vi "Chad Magic Voodoo.vi"() -> ()   [LabVIEW 2016]
panel:
  out "W trigger Y":dbl
  out "C trigger Y":dbl
  out "R trigger Y":dbl
  in  "Window Bead Trigger heights":dbl[](array[numeric])
  in  "Robot Bead Trigger heights":dbl[](array[numeric])
  in  "Center Bead Trigger heights":dbl[](array[numeric])
  out "Shutter Open":bool
  in  "Distance from\n Bead Height":dbl
  out "Recommended % Change\n in Wire Feed 1":dbl
  in  "base path":path=path "C:/Users/Mark/Desktop/BeadScan"
  in  "Write Code":bool
  out "Bead3 Size":i32
  out "Bead2 Size":i32
  out "Bead1 Size":i32
  in  "Tab Control":T1(tab)
  in  "Mark Target Bead Height":bool
  out "All Beads":cluster{dbl[], dbl[]}[](graph)
  out "Target Bead Height":dbl
  in  "Set Trigger Offset":dbl
  in  "Center Bead Corrections":dbl[](array[numeric])
  in  "Center Bead Trigger Positions":dbl[](array[numeric])
  out "Center Bead #1":cluster{dbl[], dbl[]}[](graph)
  out "Center Bead Trigger":dbl
  in  "Set Trigger Center":bool
  in  "Undo":bool
  out "Difference From Bead Height Setpoint C":dbl
  out "Recommended % Change\n in Wire Feed C":dbl
  out "Minus 5- Too lazy to math":dbl
  in  "Set Trigger Offset 2":dbl
  out "Robot Bead #2":cluster{dbl[], dbl[]}[](graph)
  in  "Robot Bead Trigger Positions":dbl[](array[numeric])
  in  "Robot Bead Corrections":dbl[](array[numeric])
  out "Robot Bead Trigger":dbl
  in  "Set Trigger Robot":bool
  in  "Undo":bool
  out "Difference From Bead Height Setpoint R":dbl
  out "Recommended % Change\n in Wire Feed R":dbl
  in  "Set Trigger Offset 3":dbl
  out "Window Bead #3":cluster{dbl[], dbl[]}[](graph)
  in  "Window Bead Trigger Positions":dbl[](array[numeric])
  in  "Window Bead Corrections":dbl[](array[numeric])
  out "Window Bead Trigger":dbl
  in  "Set Trigger Window":bool
  in  "Undo":bool
  out "Difference From Bead Height Setpoint W":dbl
  out "Recommended % Change\n in Wire Feed W":dbl
  in  "stop":bool
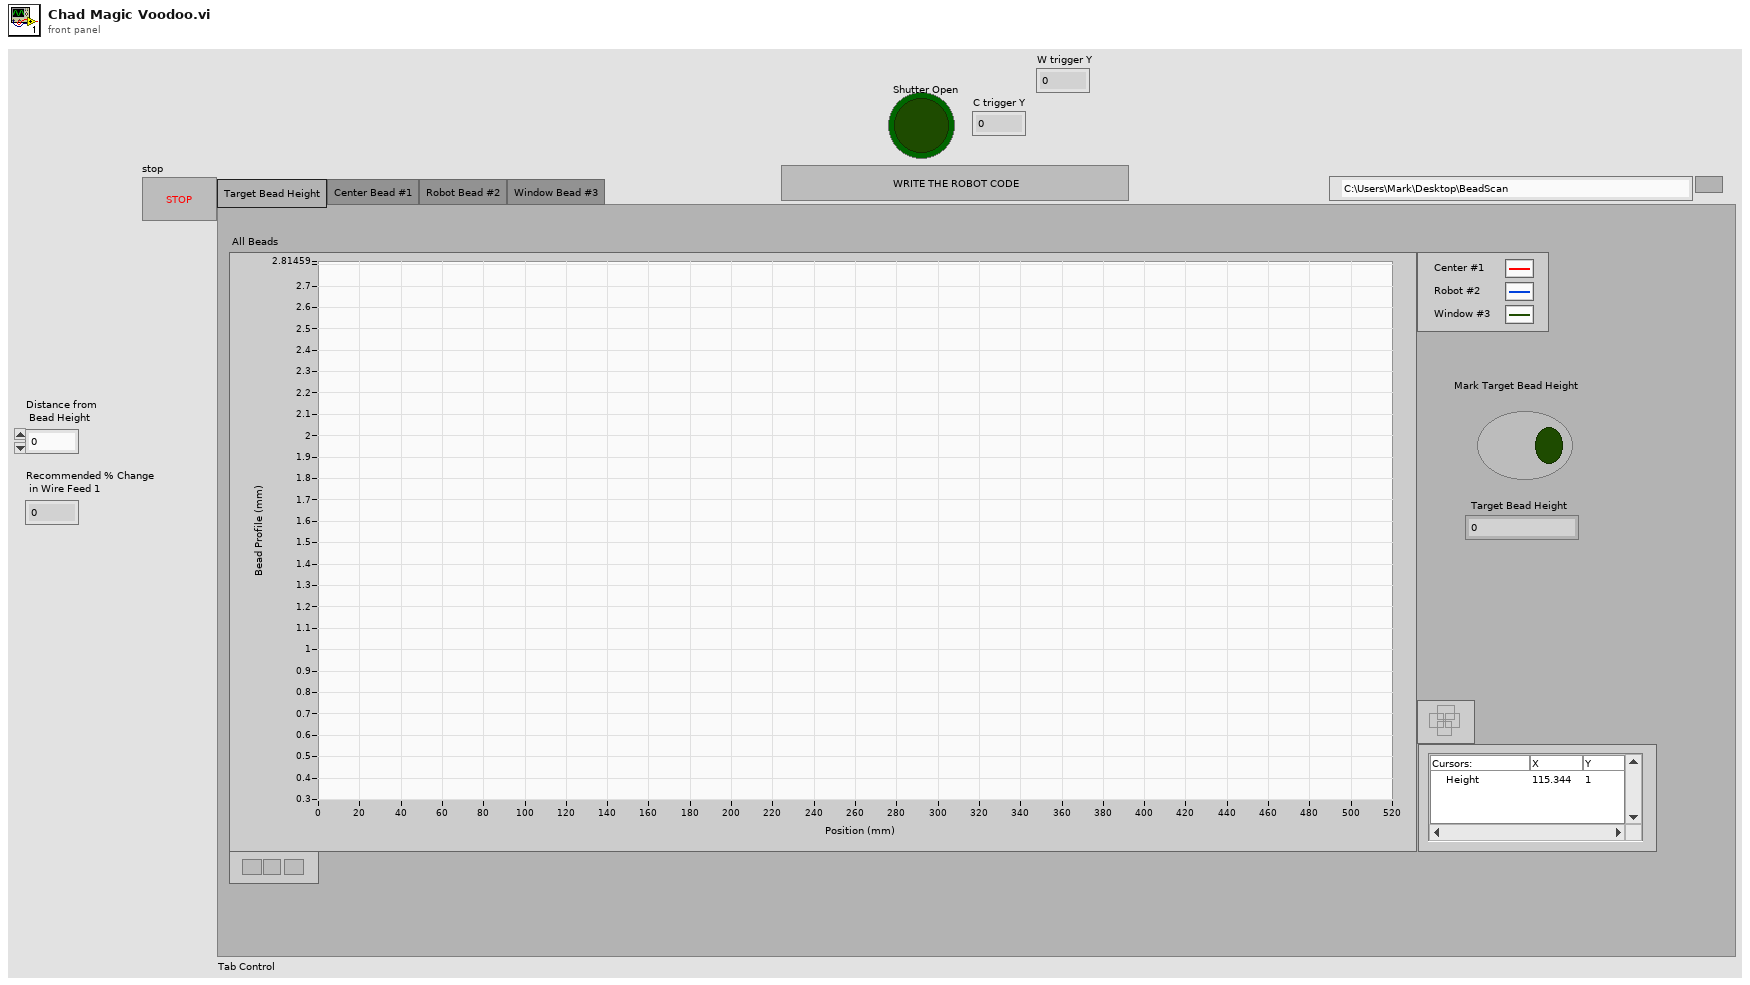
[diagram p1: front panel]
types:
  T1 = enum32{"Target Bead Height", "Center Bead #1", "Robot Bead #2", "Window Bead #3"}
  T2 = enum16{"open", "replace", "create", "open or create", "replace or create", "replace or create with confirmation"}
  T3 = cluster{"[0]":cluster{dbl[], dbl[]}, "[1]":cluster{dbl[], dbl[]}, "[2]":cluster{dbl[], dbl[]}}
  T4 = cluster{dbl[], "Center Bead Trigger heights":dbl[]}
  T5 = cluster{dbl[], "Window Bead Trigger heights":dbl[]}
  T6 = cluster{dbl[], "Robot Bead Trigger heights":dbl[]}
  T7 = cluster{dbl[], "Center Bead Trigger heights":dbl[]}[]
  T8 = cluster{dbl[], "Robot Bead Trigger heights":dbl[]}[]
  T9 = cluster{dbl[], "Window Bead Trigger heights":dbl[]}[]
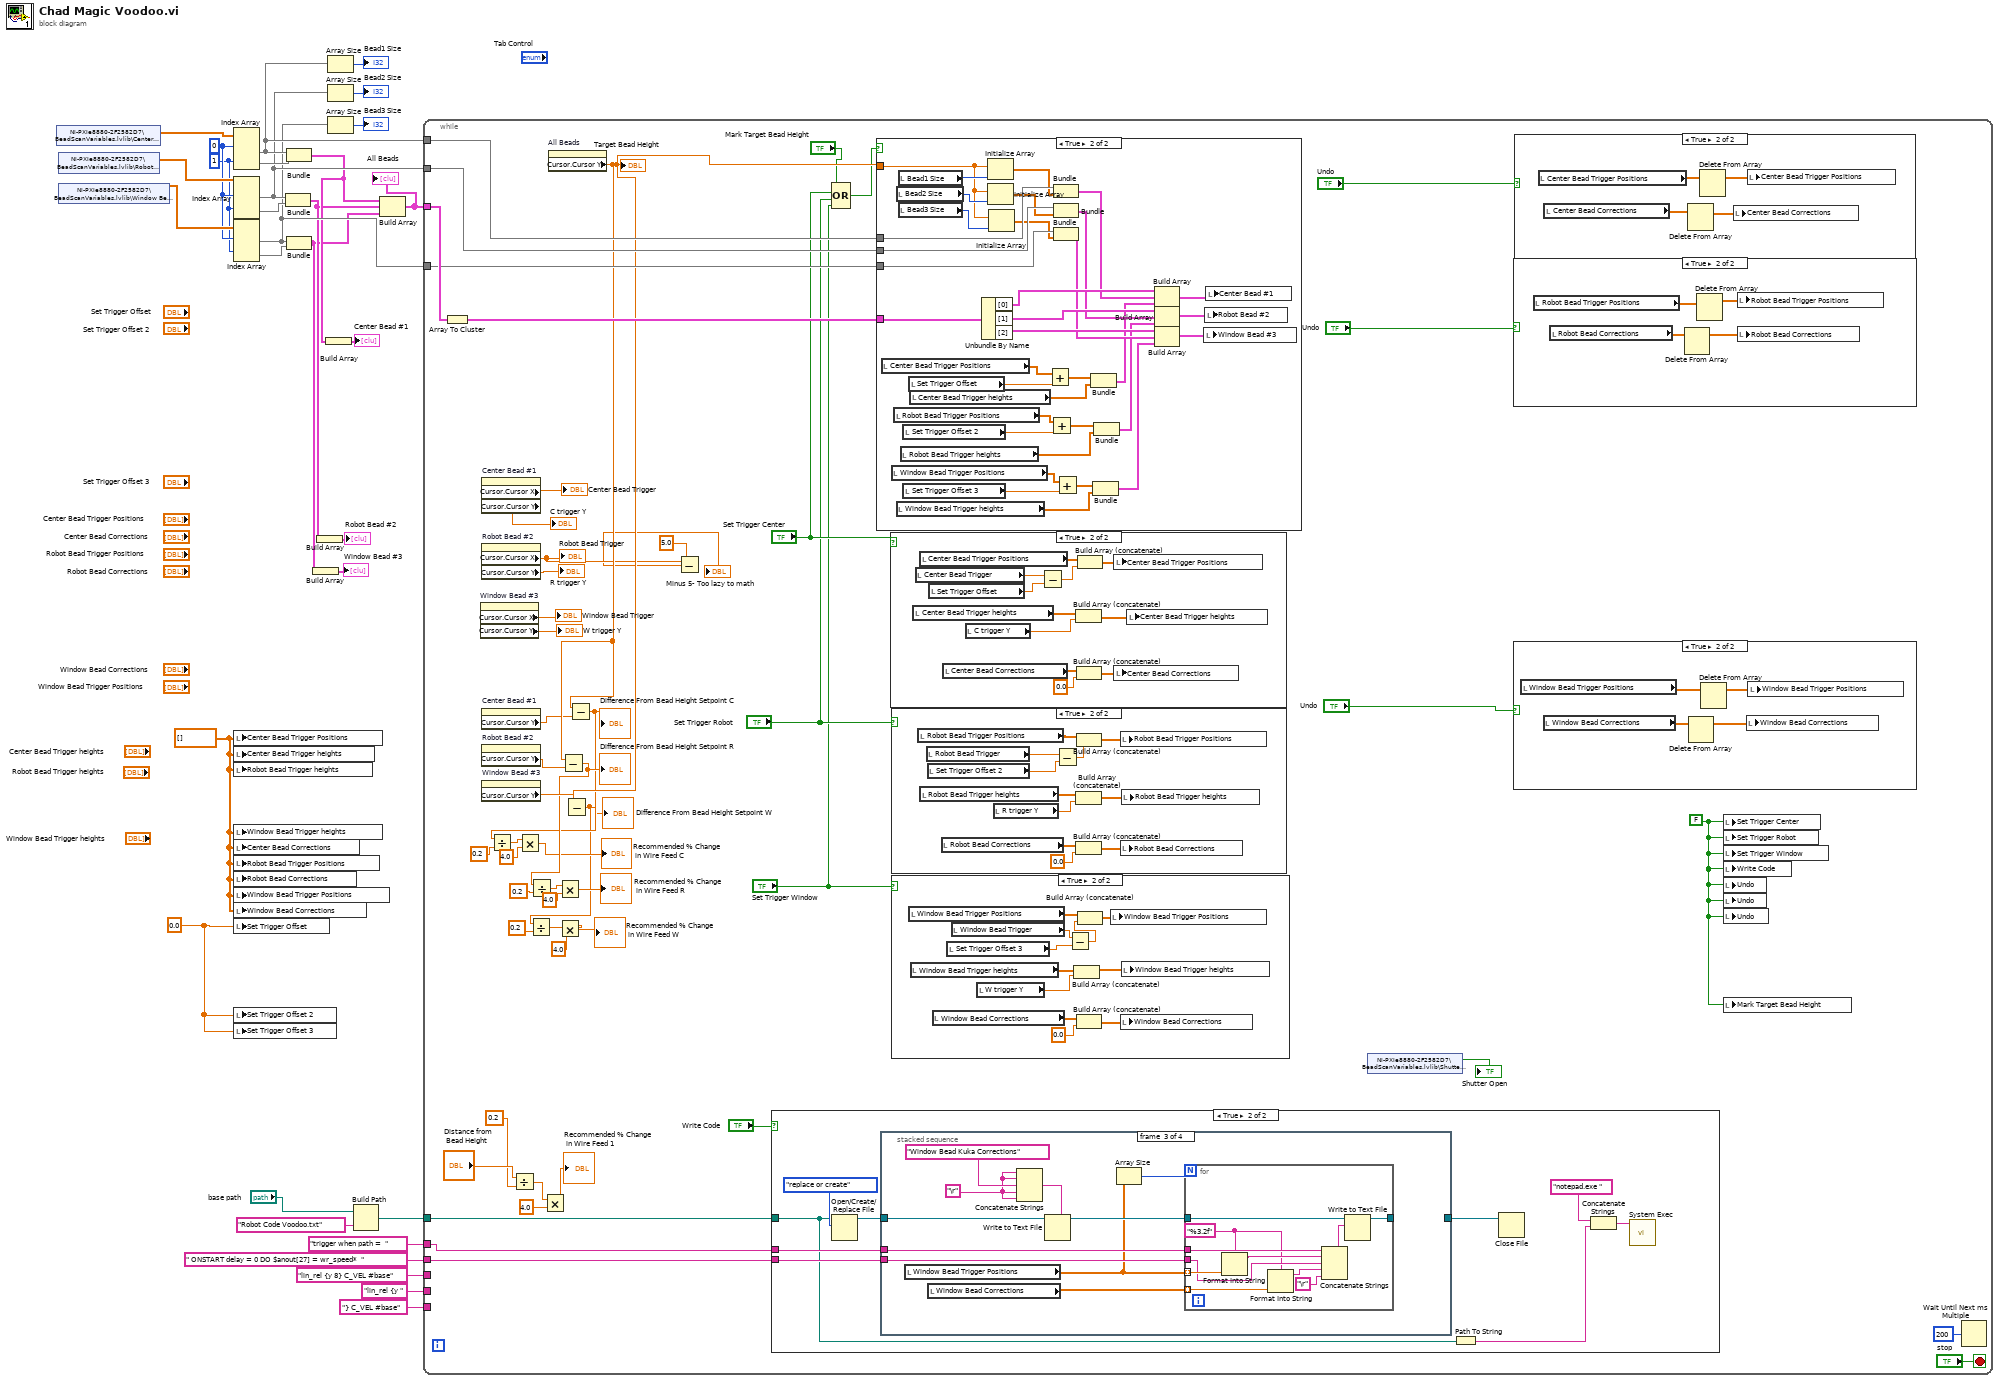
[diagram p0: block diagram]
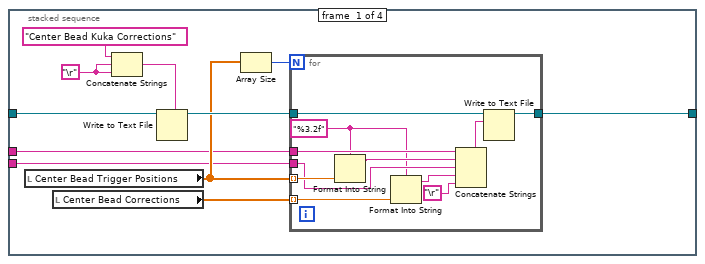
[diagram p3: hidden frame]
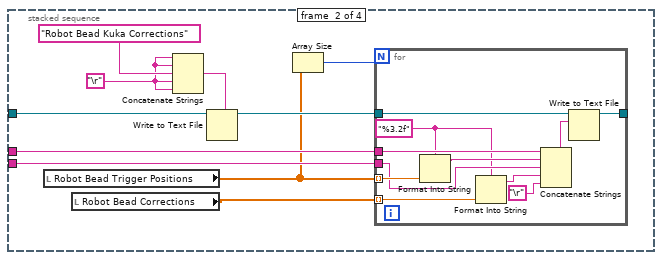
[diagram p4: hidden frame]
diagram:
  w2 = 0.0
  w1 = dbl[] []
  w26 = 1 ("index (row)")
  w27 = 0 ("index (row)")
  n1 = shared-variable "NI-PXIe8880-2F2582D7\\BeadScanVariables.lvlib\\Center Bead #1"() -> (w31:dbl[][])  [unwired: 1 in, 1 out]
  n2 = shared-variable "NI-PXIe8880-2F2582D7\\BeadScanVariables.lvlib\\Robot Bead #2"() -> (w29:dbl[][])  [unwired: 1 in, 1 out]
  n3 = shared-variable "NI-PXIe8880-2F2582D7\\BeadScanVariables.lvlib\\Window Bead #3"() -> (w28:dbl[][])  [unwired: 1 in, 1 out]
  n4 = Index Array(array=w31, index (row) #1=w27, index (row) #2=w26) -> (element #1=w19:dbl[], element #2=w30:dbl[])  [unwired: 2 in]
  n5 = Index Array(array=w29, index (row) #1=w27, index (row) #2=w26) -> (element #1=w18:dbl[], element #2=w25:dbl[])  [unwired: 2 in]
  n6 = Index Array(array=w28, index (row) #1=w27, index (row) #2=w26) -> (element #1=w17:dbl[], element #2=w24:dbl[])  [unwired: 2 in]
  n7 = local write "Center Bead Trigger Positions"(w1) -> ()
  n8 = local write "Center Bead Trigger heights"(w1) -> ()
  n9 = local write "Robot Bead Trigger heights"(w1) -> ()
  n10 = local write "Window Bead Trigger heights"(w1) -> ()
  n11 = local write "Center Bead Corrections"(w1) -> ()
  n12 = local write "Robot Bead Trigger Positions"(w1) -> ()
  n13 = local write "Robot Bead Corrections"(w1) -> ()
  n14 = local write "Window Bead Trigger Positions"(w1) -> ()
  n15 = local write "Window Bead Corrections"(w1) -> ()
  n16 = local write "Set Trigger Offset"(w2) -> ()
  n17 = local write "Set Trigger Offset 2"(w2) -> ()
  n18 = local write "Set Trigger Offset 3"(w2) -> ()
  n19 = Bundle(w18, w25) -> (w14:cluster{dbl[], dbl[]})  [unwired: 1 in]
  n20 = Bundle(w19, w30) -> (w15:cluster{dbl[], dbl[]})  [unwired: 1 in]
  n21 = Bundle(w17, w24) -> (w11:cluster{dbl[], dbl[]})  [unwired: 1 in]
  n22 = Build Array(w11) -> (→"Window Bead #3":cluster{dbl[], dbl[]}[])
  n23 = Build Array(w14) -> (→"Robot Bead #2":cluster{dbl[], dbl[]}[])
  n24 = Build Array(w15) -> (→"Center Bead #1":cluster{dbl[], dbl[]}[])
  n25 = Array Size(array=w19) -> (size(s)=→"Bead1 Size":i32)
  n26 = Array Size(array=w18) -> (size(s)=→"Bead2 Size":i32)
  n27 = Array Size(array=w17) -> (size(s)=→"Bead3 Size":i32)
  n28 = Build Path(base path="base path", name or relative path="Robot Code Voodoo.txt") -> (appended path=w8:path)
  n29 = Build Array(w15, w14, w11) -> (w20:cluster{dbl[], dbl[]}[])
  "All Beads" <- w20
  n30 = while {
    tunnel: w20 -> [w81]
    tunnel: w19 -> [w79]
    tunnel: w18 -> [w78]
    tunnel: w17 -> [w77]
    tunnel: w8 -> [w72]
    tunnel: "trigger when path =  " -> [w71]
    tunnel: " ONSTART delay = 0 DO $anout[27] = wr_speed*  " -> [w70]
    tunnel: "lin_rel {y 8} C_VEL #base" -> [_]
    tunnel: "lin_rel {y " -> [_]
    tunnel: "} C_VEL #base" -> [_]
    stop <- "stop" stop-if-true
    w69 = FALSE
    n31 = Array To Cluster(array=w81) -> (cluster=w80:T3)
    n32 = property on="Window Bead #3" class="XYGraph (strict)"() -> ("Cursor.Cursor X"=→"Window Bead Trigger":dbl, "Cursor.Cursor Y"=→"W trigger Y":dbl)  [unwired: 2 in, 2 out]
    n33 = property on="Center Bead #1" class="XYGraph (strict)"() -> ("Cursor.Cursor X"=→"Center Bead Trigger":dbl, "Cursor.Cursor Y"=→"C trigger Y":dbl)  [unwired: 2 in, 2 out]
    n34 = property on="Robot Bead #2" class="XYGraph (strict)"() -> ("Cursor.Cursor X"=w34:dbl, "Cursor.Cursor Y"=→"R trigger Y":dbl)  [unwired: 2 in, 2 out]
    "Robot Bead Trigger" <- w34
    n35 = property on="Center Bead #1" class="XYGraph (strict)"() -> ("Cursor.Cursor Y"=w61:dbl)  [unwired: 2 in, 2 out]
    n36 = property on="Robot Bead #2" class="XYGraph (strict)"() -> ("Cursor.Cursor Y"=w60:dbl)  [unwired: 2 in, 2 out]
    n37 = property on="Window Bead #3" class="XYGraph (strict)"() -> ("Cursor.Cursor Y"=w59:dbl)  [unwired: 2 in, 2 out]
    n38 = Divide(x="Distance from\n Bead Height", y=0.2) -> (x/y=w66:dbl)
    n39 = Multiply(x=w66, y=4.0) -> (x*y=→"Recommended % Change\n in Wire Feed 1":dbl)
    n40 = property on="All Beads" class="XYGraph (strict)"() -> ("Cursor.Cursor Y"=w62:dbl)  [unwired: 2 in, 2 out]
    "Target Bead Height" <- w62
    n41 = Subtract(x=w62, y=w60) -> (x-y=w42:dbl)
    "Difference From Bead Height Setpoint R" <- w42
    n42 = Divide(x=w42, y=0.2) -> (x/y=w48:dbl)
    n43 = Multiply(x=w48, y=4.0) -> (x*y=→"Recommended % Change\n in Wire Feed R":dbl)
    n44 = Subtract(x=w62, y=w59) -> (x-y=w35:dbl)
    "Difference From Bead Height Setpoint W" <- w35
    n45 = Divide(x=w35, y=0.2) -> (x/y=w45:dbl)
    n46 = Multiply(x=w45, y=4.0) -> (x*y=→"Recommended % Change\n in Wire Feed W":dbl)
    n47 = Subtract(x=w62, y=w61) -> (x-y=w37:dbl)
    "Difference From Bead Height Setpoint C" <- w37
    n48 = Divide(x=w37, y=0.2) -> (x/y=w40:dbl)
    n49 = Multiply(x=w40, y=4.0) -> (x*y=→"Recommended % Change\n in Wire Feed C":dbl)
    n50 = Subtract(x=w34, y=5.0) -> (x-y=→"Minus 5- Too lazy to math":dbl)
    n51 = case shown="True" "Write Code" {
      tunnel: w72 -> [_ w85]
      tunnel: w71 -> [_ w92]
      tunnel: w70 -> [_ w91]
      frame False {
      }
      frame True {
        n52 = Open/Create/Replace File(file path (use dialog)=w85, operation (0:open)=T2."replace or create") -> (refnum out=w93:refnum<file>)  [unwired: 4 in, 2 out]
        n53 = stacked-sequence {
          tunnel: w93 -> [w101 w122 w143 _]
          tunnel: w92 -> [w96 w120 w141 _]
          tunnel: w91 -> [w95 w119 w140 _]
          tunnel: [w94 _ _ _] -> w90
          frame #0 {
            w103 = "\r"
            n54 = local read "Center Bead Trigger Positions"() -> (w98:dbl[])
            n55 = local read "Center Bead Corrections"() -> (w97:dbl[])
            n56 = Concatenate Strings("Center Bead Kuka Corrections", w103, w103) -> (w102:string)
            n57 = Write to Text File(file (use dialog)=w101, text=w102) -> (refnum out=w100:refnum<file>)  [unwired: 2 in, 2 out]
            n58 = Array Size(array=w98) -> (size(s)=w99:i32)
            n59 = for {
              N: w99 -> [_]
              tunnel: w100 -> [w115]
              tunnel: w98 -> [w112] mode=indexing
              tunnel: w97 -> [w109] mode=indexing
              tunnel: w96 -> [w114]
              tunnel: w95 -> [w110]
              tunnel: [w107] -> w94
              w106 = "%3.2f" ("format string")
              n60 = Format Into String(format string=w106, w112) -> (resulting string=w113:string)  [unwired: 2 in, 1 out]
              n61 = Format Into String(format string=w106, w109) -> (resulting string=w108:string)  [unwired: 2 in, 1 out]
              n62 = Concatenate Strings(w114, w113, w110, w108, "\r") -> (w111:string)
              n63 = Write to Text File(file (use dialog)=w115, text=w111) -> (refnum out=w107:refnum<file>)  [unwired: 2 in, 2 out]
            }
          }
          frame #1 {
            w116 = "\r"
            n64 = local read "Robot Bead Trigger Positions"() -> (w117:dbl[])
            n65 = local read "Robot Bead Corrections"() -> (w118:dbl[])
            n66 = Concatenate Strings(w116, w116, "Robot Bead Kuka Corrections", w116, w116) -> (w124:string)
            n67 = Write to Text File(file (use dialog)=w122, text=w124) -> (refnum out=w123:refnum<file>)  [unwired: 2 in, 2 out]
            n68 = Array Size(array=w117) -> (size(s)=w121:i32)
            n69 = for {
              N: w121 -> [_]
              tunnel: w123 -> [w136]
              tunnel: w117 -> [w133] mode=indexing
              tunnel: w118 -> [w130] mode=indexing
              tunnel: w120 -> [w135]
              tunnel: w119 -> [w131]
              tunnel: [w128] -> _
              w127 = "%3.2f" ("format string")
              n70 = Format Into String(format string=w127, w133) -> (resulting string=w134:string)  [unwired: 2 in, 1 out]
              n71 = Format Into String(format string=w127, w130) -> (resulting string=w129:string)  [unwired: 2 in, 1 out]
              n72 = Concatenate Strings(w135, w134, w131, w129, "\r") -> (w132:string)
              n73 = Write to Text File(file (use dialog)=w136, text=w132) -> (refnum out=w128:refnum<file>)  [unwired: 2 in, 2 out]
            }
          }
          frame #2 {
            w137 = "\r"
            n74 = local read "Window Bead Trigger Positions"() -> (w138:dbl[])
            n75 = local read "Window Bead Corrections"() -> (w139:dbl[])
            n76 = Concatenate Strings(w137, w137, "Window Bead Kuka Corrections", w137, w137) -> (w145:string)
            n77 = Write to Text File(file (use dialog)=w143, text=w145) -> (refnum out=w144:refnum<file>)  [unwired: 2 in, 2 out]
            n78 = Array Size(array=w138) -> (size(s)=w142:i32)
            n79 = for {
              N: w142 -> [_]
              tunnel: w144 -> [w157]
              tunnel: w138 -> [w154] mode=indexing
              tunnel: w139 -> [w151] mode=indexing
              tunnel: w141 -> [w156]
              tunnel: w140 -> [w152]
              tunnel: [w149] -> _
              w148 = "%3.2f" ("format string")
              n80 = Format Into String(format string=w148, w154) -> (resulting string=w155:string)  [unwired: 2 in, 1 out]
              n81 = Format Into String(format string=w148, w151) -> (resulting string=w150:string)  [unwired: 2 in, 1 out]
              n82 = Concatenate Strings(w156, w155, w152, w150, "\r") -> (w153:string)
              n83 = Write to Text File(file (use dialog)=w157, text=w153) -> (refnum out=w149:refnum<file>)  [unwired: 2 in, 2 out]
            }
          }
          frame #3 {
          }
        }
        n84 = Path To String(path=w85) -> (string=w86:string)
        n85 = Close File(refnum=w90) -> ()  [unwired: 1 in, 2 out]
        n86 = Concatenate Strings("notepad.exe " ("command line"), w86) -> (w88:string)
        n87 = call <vilib>:"System Exec.vi"("command line"=w88) -> ()  [unwired: 7 in, 4 out]
      }
    }
    n88 = Compound Arithmetic op=OR("Mark Target Bead Height", "Set Trigger Center", "Set Trigger Robot", "Set Trigger Window") -> (w53:bool)
    n89 = case shown="True" w53 {
      tunnel: w62 -> [_ w235]
      tunnel: w80 -> [_ w233]
      tunnel: w79 -> [_ w232]
      tunnel: w78 -> [_ w230]
      tunnel: w77 -> [_ w229]
      frame False {
      }
      frame True {
        n90 = local read "Center Bead Trigger Positions"() -> (w213:dbl[])
        n91 = local read "Window Bead Trigger Positions"() -> (w207:dbl[])
        n92 = local read "Robot Bead Trigger Positions"() -> (w210:dbl[])
        n93 = local read "Bead2 Size"() -> (w236:i32)
        n94 = local read "Window Bead Trigger heights"() -> (w206:dbl[])
        n95 = local read "Bead1 Size"() -> (w237:i32)
        n96 = local read "Bead3 Size"() -> (w234:i32)
        n97 = local read "Robot Bead Trigger heights"() -> (w208:dbl[])
        n98 = local read "Set Trigger Offset 2"() -> (w216:dbl)
        n99 = local read "Set Trigger Offset 3"() -> (w215:dbl)
        n100 = local read "Set Trigger Offset"() -> (w217:dbl)
        n101 = local read "Center Bead Trigger heights"() -> (w211:dbl[])
        n102 = Unbundle By Name(w233) -> ("[0]"=w226:cluster{dbl[], dbl[]}, "[1]"=w224:cluster{dbl[], dbl[]}, "[2]"=w222:cluster{dbl[], dbl[]})
        n103 = Initialize Array(w235, w237) -> (w231:dbl[])
        n104 = Initialize Array(w235, w236) -> (w227:dbl[])
        n105 = Initialize Array(w235, w234) -> (w228:dbl[])
        n106 = Add(x=w213, y=w217) -> (x+y=w212:dbl[])
        n107 = Add(x=w210, y=w216) -> (x+y=w209:dbl[])
        n108 = Bundle(w232, w231) -> (w225:cluster{dbl[], dbl[]})  [unwired: 1 in]
        n109 = Bundle(w230, w227) -> (w223:cluster{dbl[], dbl[]})  [unwired: 1 in]
        n110 = Bundle(w229, w228) -> (w221:cluster{dbl[], dbl[]})  [unwired: 1 in]
        n111 = Add(x=w207, y=w215) -> (x+y=w214:dbl[])
        n112 = Bundle(w212, "Center Bead Trigger heights"=w211) -> (w205:T4)  [unwired: 1 in]
        n113 = Bundle(w214, "Window Bead Trigger heights"=w206) -> (w203:T5)  [unwired: 1 in]
        n114 = Bundle(w209, "Robot Bead Trigger heights"=w208) -> (w204:T6)  [unwired: 1 in]
        n115 = Build Array(w226, w225, w205) -> (w220:T7)
        n116 = Build Array(w224, w223, w204) -> (w219:T8)
        n117 = Build Array(w222, w221, w203) -> (w218:T9)
        n118 = local write "Window Bead #3"(w218) -> ()
        n119 = local write "Robot Bead #2"(w219) -> ()
        n120 = local write "Center Bead #1"(w220) -> ()
      }
    }
    n121 = case shown="True" "Set Trigger Center" {
      frame False {
      }
      frame True {
        n122 = local read "Center Bead Trigger heights"() -> (w194:dbl[])
        n123 = local read "Center Bead Trigger"() -> (w197:dbl)
        n124 = local read "Center Bead Trigger Positions"() -> (w202:dbl[])
        n125 = local read "Set Trigger Offset"() -> (w195:dbl)
        n126 = local read "Center Bead Corrections"() -> (w200:dbl[])
        n127 = local read "C trigger Y"() -> (w193:dbl)
        n128 = Subtract(x=w197, y=w195) -> (x-y=w196:dbl)
        n129 = Build Array (concatenate)(w194, w193) -> (w192:dbl[])
        n130 = Build Array (concatenate)(w200, 0.0) -> (w198:dbl[])
        n131 = Build Array (concatenate)(w202, w196) -> (w201:dbl[])
        n132 = local write "Center Bead Trigger Positions"(w201) -> ()
        n133 = local write "Center Bead Corrections"(w198) -> ()
        n134 = local write "Center Bead Trigger heights"(w192) -> ()
      }
    }
    n135 = case shown="True" "Set Trigger Robot" {
      frame False {
      }
      frame True {
        n136 = local read "Robot Bead Trigger Positions"() -> (w189:dbl[])
        n137 = local read "Robot Bead Trigger heights"() -> (w182:dbl[])
        n138 = local read "Robot Bead Trigger"() -> (w186:dbl)
        n139 = local read "Set Trigger Offset 2"() -> (w184:dbl)
        n140 = local read "Robot Bead Corrections"() -> (w191:dbl[])
        n141 = local read "R trigger Y"() -> (w181:dbl)
        n142 = Subtract(x=w186, y=w184) -> (x-y=w185:dbl)
        n143 = Build Array (concatenate)(w182, w181) -> (w183:dbl[])
        n144 = Build Array (concatenate)(w191, 0.0) -> (w187:dbl[])
        n145 = Build Array (concatenate)(w189, w185) -> (w188:dbl[])
        n146 = local write "Robot Bead Trigger Positions"(w188) -> ()
        n147 = local write "Robot Bead Corrections"(w187) -> ()
        n148 = local write "Robot Bead Trigger heights"(w183) -> ()
      }
    }
    n149 = case shown="True" "Set Trigger Window" {
      frame False {
      }
      frame True {
        n150 = local read "Window Bead Trigger Positions"() -> (w179:dbl[])
        n151 = local read "Window Bead Trigger heights"() -> (w172:dbl[])
        n152 = local read "Window Bead Corrections"() -> (w178:dbl[])
        n153 = local read "Set Trigger Offset 3"() -> (w175:dbl)
        n154 = local read "Window Bead Trigger"() -> (w174:dbl)
        n155 = local read "W trigger Y"() -> (w171:dbl)
        n156 = Subtract(x=w174, y=w175) -> (x-y=w173:dbl)
        n157 = Build Array (concatenate)(w172, w171) -> (w170:dbl[])
        n158 = Build Array (concatenate)(w178, 0.0) -> (w176:dbl[])
        n159 = Build Array (concatenate)(w179, w173) -> (w177:dbl[])
        n160 = local write "Window Bead Trigger Positions"(w177) -> ()
        n161 = local write "Window Bead Corrections"(w176) -> ()
        n162 = local write "Window Bead Trigger heights"(w170) -> ()
      }
    }
    n163 = shared-variable "NI-PXIe8880-2F2582D7\\BeadScanVariables.lvlib\\Shutter Open"() -> (→"Shutter Open":bool)  [unwired: 1 in, 1 out]
    n164 = case shown="True" "Undo" {
      frame False {
      }
      frame True {
        n165 = local read "Robot Bead Trigger Positions"() -> (w164:dbl[])
        n166 = local read "Robot Bead Corrections"() -> (w165:dbl[])
        n167 = Delete From Array(array=w165) -> (array with subset deleted=w162:dbl[])  [unwired: 2 in, 1 out]
        n168 = Delete From Array(array=w164) -> (array with subset deleted=w163:dbl[])  [unwired: 2 in, 1 out]
        n169 = local write "Robot Bead Trigger Positions"(w163) -> ()
        n170 = local write "Robot Bead Corrections"(w162) -> ()
      }
    }
    n171 = case shown="True" "Undo" {
      frame False {
      }
      frame True {
        n172 = local read "Window Bead Trigger Positions"() -> (w160:dbl[])
        n173 = local read "Window Bead Corrections"() -> (w159:dbl[])
        n174 = Delete From Array(array=w159) -> (array with subset deleted=w158:dbl[])  [unwired: 2 in, 1 out]
        n175 = Delete From Array(array=w160) -> (array with subset deleted=w161:dbl[])  [unwired: 2 in, 1 out]
        n176 = local write "Window Bead Corrections"(w158) -> ()
        n177 = local write "Window Bead Trigger Positions"(w161) -> ()
      }
    }
    n178 = case shown="True" "Undo" {
      frame False {
      }
      frame True {
        n179 = local read "Center Bead Trigger Positions"() -> (w168:dbl[])
        n180 = local read "Center Bead Corrections"() -> (w167:dbl[])
        n181 = Delete From Array(array=w167) -> (array with subset deleted=w166:dbl[])  [unwired: 2 in, 1 out]
        n182 = Delete From Array(array=w168) -> (array with subset deleted=w169:dbl[])  [unwired: 2 in, 1 out]
        n183 = local write "Center Bead Corrections"(w166) -> ()
        n184 = local write "Center Bead Trigger Positions"(w169) -> ()
      }
    }
    n185 = local write "Set Trigger Center"(w69) -> ()
    n186 = local write "Set Trigger Robot"(w69) -> ()
    n187 = local write "Set Trigger Window"(w69) -> ()
    n188 = local write "Write Code"(w69) -> ()
    n189 = local write "Undo"(w69) -> ()
    n190 = local write "Undo"(w69) -> ()
    n191 = local write "Undo"(w69) -> ()
    n192 = local write "Mark Target Bead Height"(w69) -> ()
    n193 = Wait Until Next ms Multiple(millisecond multiple=u32 200) -> ()  [unwired: 1 out]
  }
